vi "HomeWorkReadAndWriteToFile.vi"   [LabVIEW 2018]
types:
  T1 = enum16{"open", "replace", "create", "open or create", "replace or create", "replace or create with confirmation"}
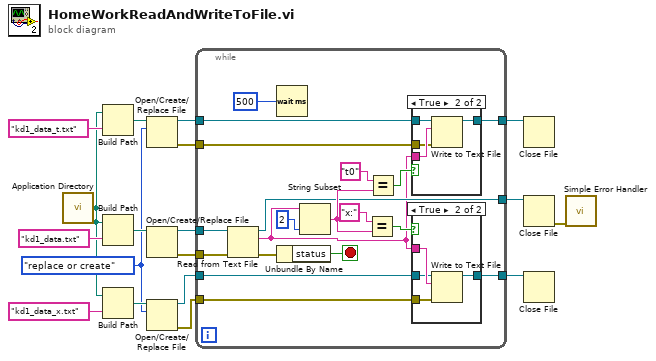
[diagram p0: block diagram]
diagram:
  w1 = T1."replace or create" ("operation (0:open)")
  n1 = call <vilib>:"Application Directory.vi"() -> ("Application Directory"=w2:path)
  n2 = Build Path(base path=w2, name or relative path="kd1_data_t.txt") -> (appended path=w6:path)
  n3 = Build Path(base path=w2, name or relative path="kd1_data.txt") -> (appended path=w8:path)
  n4 = Build Path(base path=w2, name or relative path="kd1_data_x.txt") -> (appended path=w7:path)
  n5 = Open/Create/Replace File(file path (use dialog)=w6, operation (0:open)=w1) -> (refnum out=w10:refnum<file>, error out=w9:errorcluster)  [unwired: 4 in, 1 out]
  n6 = Open/Create/Replace File(file path (use dialog)=w8) -> (refnum out=w13:refnum<file>, error out=w14:errorcluster)  [unwired: 5 in, 1 out]
  n7 = Open/Create/Replace File(file path (use dialog)=w7, operation (0:open)=w1) -> (refnum out=w12:refnum<file>, error out=w11:errorcluster)  [unwired: 4 in, 1 out]
  n8 = while {
    tunnel: [w29] -> w17
    tunnel: [w28] -> w16
    tunnel: [w27] -> w15
    tunnel: w14 -> [w25]
    tunnel: w13 -> [w24]
    tunnel: w12 -> [w23]
    tunnel: w11 -> [w22]
    tunnel: w10 -> [w21]
    tunnel: w9 -> [w20]
    stop <- w31 stop-if-true
    n9 = Read from Text File(file (use dialog)=w24, error in=w25) -> (refnum out=w29:refnum<file>, text=w26:string, error out=w30:errorcluster)  [unwired: 2 in, 1 out]
    n10 = Wait (ms)(milliseconds to wait=500) -> ()  [unwired: 1 out]
    n11 = Unbundle By Name(w30) -> ("status"=w31:bool)
    n12 = String Subset(string=w26, length (rest)=2 ("length (rest)")) -> (substring=w35:string)  [unwired: 1 in]
    n13 = Equal?(x="x:", y=w35) -> (x = y?=w32:bool)
    n14 = Equal?(x="t0", y=w35) -> (x = y?=w33:bool)
    n15 = case shown="True" w33 {
      tunnel: [w38 w42] -> w28
      tunnel: w26 -> [_ w41]
      tunnel: w21 -> [w38 w40]
      tunnel: w20 -> [_ w39]
      frame False {
      }
      frame True {
        n16 = Write to Text File(file (use dialog)=w40, text=w41, error in=w39) -> (refnum out=w42:refnum<file>)  [unwired: 1 in, 2 out]
      }
    }
    n17 = case shown="True" w32 {
      tunnel: [w43 w47] -> w27
      tunnel: w26 -> [_ w46]
      tunnel: w23 -> [w43 w45]
      tunnel: w22 -> [_ w44]
      frame False {
      }
      frame True {
        n18 = Write to Text File(file (use dialog)=w45, text=w46, error in=w44) -> (refnum out=w47:refnum<file>)  [unwired: 1 in, 2 out]
      }
    }
  }
  n19 = Close File(refnum=w16) -> ()  [unwired: 1 in, 2 out]
  n20 = Close File(refnum=w17) -> (error out=w18:errorcluster)  [unwired: 1 in, 1 out]
  n21 = Close File(refnum=w15) -> ()  [unwired: 1 in, 2 out]
  n22 = call <vilib>:"Simple Error Handler.vi"("error in (no error)"=w18) -> ()  [unwired: 4 in, 5 out]
